vi "CHECK 20TVTI QUEUE.vi"(7 "error in (no error)":errorcluster, 10 "queue":refnum<queue>) -> (0 "error out":errorcluster, 1 "VTI Control":T1, 3 "New Entries?":bool)   [LabVIEW 2019]
uses:
  Gustav/20TVTI_Control.ctl
panel:
  out "Numeric":i32
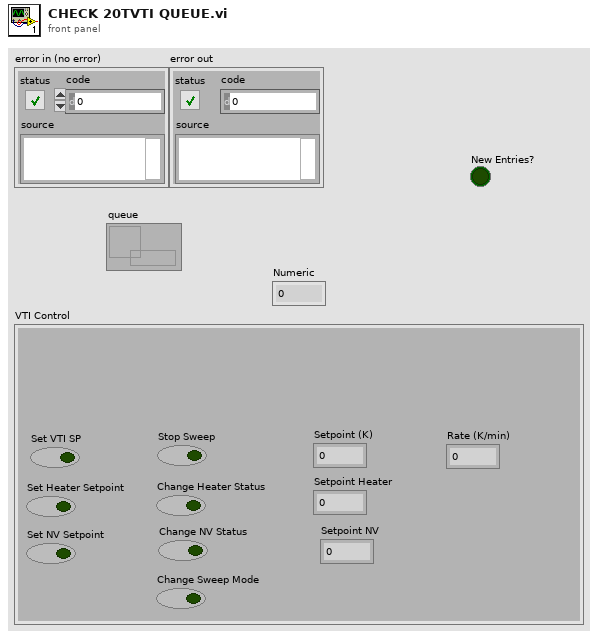
[diagram p1: front panel]
types:
  T1 = typedef "20TVTI_Control.ctl" = cluster{"Set VTI SP":bool, "Change NV Status":bool, "Set NV Setpoint":bool, "Change Heater Status":bool, "Set Heater Setpoint":bool, "Stop Sweep":bool, "Setpoint (K)":dbl, "Rate (K/min)":dbl, "Setpoint Heater":dbl, "Setpoint NV":dbl, "Change Sweep Mode":bool}
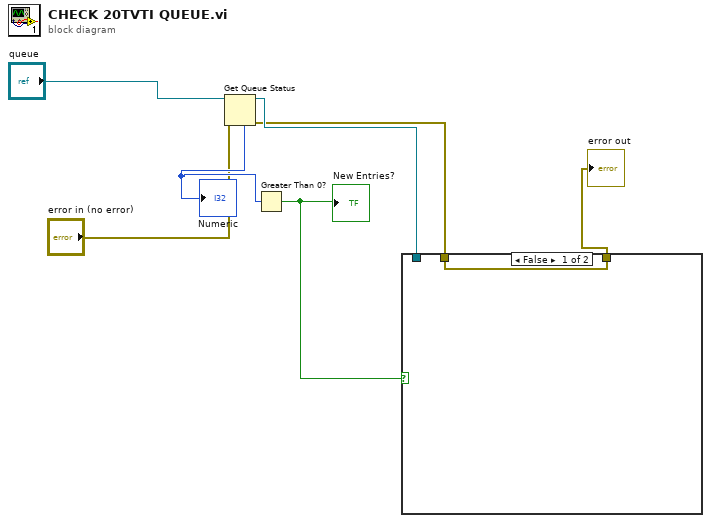
[diagram p0: block diagram]
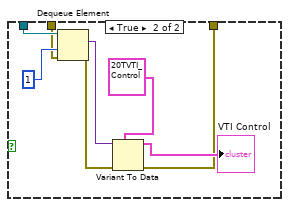
[diagram p2: hidden frame]
diagram:
  n1 = Get Queue Status(queue="queue", error in (no error)="error in (no error)") -> (queue out=w6:refnum<queue>, error out=w3:errorcluster, # elements in queue=w7:i32)  [unwired: 1 in, 5 out]
  "Numeric" <- w7
  n2 = Greater Than 0?(x=w7) -> (x > 0?=w4:bool)
  "New Entries?" <- w4
  n3 = case shown="False" w4 {
    tunnel: w6 -> [_ w13]
    tunnel: w3 -> [w8 w11]
    tunnel: [w8 w9] -> w1
    frame False {
    }
    frame True {
      n4 = Dequeue Element(queue=w13, timeout in ms (-1)=1, error in (no error)=w11) -> (element=w15:variant, error out=w10:errorcluster)  [unwired: 2 out]
      n5 = Variant To Data(error in=w10, type=T1 {"Set VTI SP"=TRUE, "Change NV Status"=TRUE, "Set NV Setpoint"=TRUE, "Change Heater Status"=FALSE, "Set Heater Setpoint"=FALSE, "Stop Sweep"=FALSE, "Setpoint (K)"=0.0, "Rate (K/min)"=0.0, "Setpoint Heater"=0.0, "Setpoint NV"=0.0, "Change Sweep Mode"=FALSE} ("Cluster 3"), Variant=w15) -> (data=→"VTI Control":T1, error out=w9:errorcluster)
    }
  }
  "error out" <- w1
